vi "PJT_15.vi"() -> ()   [LabVIEW 2019]
panel:
  in  "정지":bool
  out "미터":dbl(knob) scale=0.0..10.0
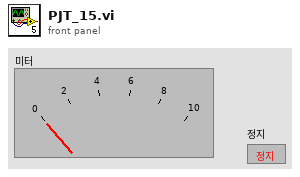
[diagram p1: front panel]
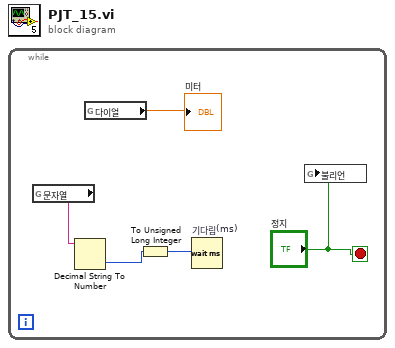
[diagram p0: block diagram]
diagram:
  n1 = while {
    stop <- "정지" stop-if-true
    n2 = global read "글로벌 1.vi" "문자열"() -> (w4:string)
    n3 = Decimal String To Number(string=w4) -> (number=w3:i32)  [unwired: 2 in, 1 out]
    n4 = global read "글로벌 1.vi" "다이얼"() -> (→"미터":dbl)
    n5 = To Unsigned Long Integer(number=w3) -> (unsigned 32bit integer=w2:u32)
    n6 = Wait (ms) "기다림(ms)"(milliseconds to wait=w2) -> ()  [unwired: 1 out]
    n7 = global write "글로벌 1.vi" "불리언"("정지") -> ()
  }
